vi "Event-Display.vi"(7 "Display":T1(ring), 8 "error in (no error)":errorcluster, 10 "Data ref. in":refnum<data-value>, 11 "UI ref. in":refnum<data-value>) -> (0 "error out":errorcluster, 2 "Data ref.":refnum<data-value>, 3 "UI ref.":refnum<data-value>)   [LabVIEW 2013, in "CameraVision.lvlib" / "CV-UI.lvclass"]
uses:
  CV-UI.lvclass
  Main/CV-Main.lvclass
  CV-UI.lvclass/CV-UI.ctl
  Main/Main-actions.ctl
  Read Display-tab.vi
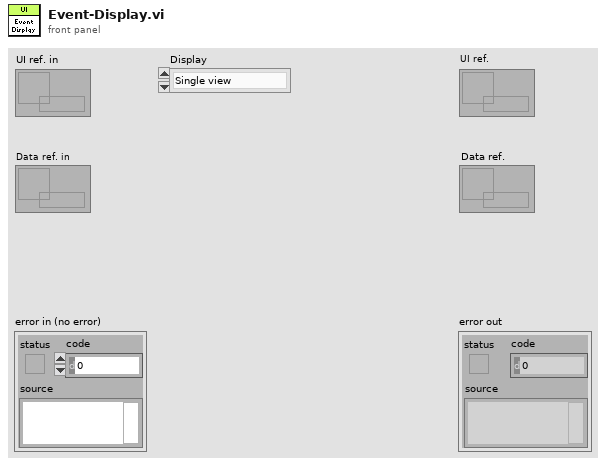
[diagram p1: front panel]
types:
  T1 = enum32{"Single view", "Dual view", "Analysis", "History", "Temperature field", "Mapping", "Debug"}
  T2 = typedef "CameraVision.lvlib/CV-Main.lvclass/Main-actions.ctl" = enum16{"Idle", "Initialize", "Load defaults", "Update settings", "Check settings", "Save settings", "Save settings with dialog", "Load settings", "Load data", "Activate", "Start", "Wait for start signal", "Acquire & process", "Iterate", "Stop", "Refresh display", "Refresh status", "View camera settings", "View grabber settings", "Exit"}
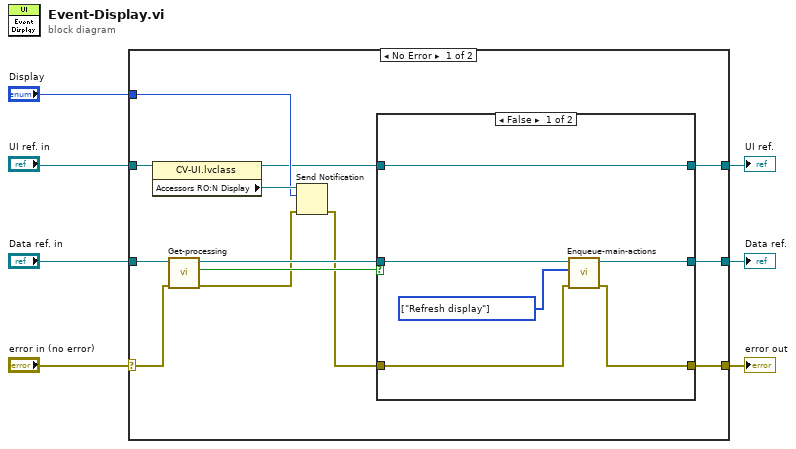
[diagram p0: block diagram]
diagram:
  n1 = case shown="No Error" "error in (no error)" {
    selector: "error in (no error)" -> [w15 w32]
    tunnel: [w14 w32] -> w6
    tunnel: [w17 w31] -> w4
    tunnel: "UI ref. in" -> [w13 w31]
    tunnel: "Data ref. in" -> [w20 w30]
    tunnel: "Display" -> [w9 _]
    tunnel: [w16 w30] -> w2
    frame No Error {
      n2 = property class="CV-UI.lvclass"(reference=w13) -> (reference out=w8:refnum<data-value>, "Accessors RO:N Display"=w12:refnum<notifier>)  [unwired: 1 in, 1 out]
      n3 = call "Get-processing.vi"("error in (no error)"=w15, "Data ref. in"=w20) -> ("error out"=w11:errorcluster, "Processing?"=w18:bool, "Data ref."=w19:refnum<data-value>)  [unwired: 7 in]
      n4 = Send Notification(notification=w9, notifier=w12, error in (no error)=w11) -> (error out=w10:errorcluster)  [unwired: 1 out]
      n5 = case shown="False" w18 {
        tunnel: w8 -> [w23 w28]
        tunnel: w19 -> [w22 w27]
        tunnel: [w23 w28] -> w17
        tunnel: [w21 w27] -> w16
        tunnel: w10 -> [w25 w29]
        tunnel: [w24 w29] -> w14
        frame False {
          w26 = T2[] [enum."Refresh display"] items=["Idle", "Initialize", "Load defaults", "Update settings", "Check settings", "Save settings", "Save settings with dialog", "Load settings", "Load data", "Activate", "Start", "Wait for start signal", "Acquire & process", "Iterate", "Stop", "Refresh display", "Refresh status", "View camera settings", "View grabber settings", "Exit"] ("State array")
          n6 = call "Enqueue-main-actions.vi"("error in (no error)"=w25, "State array"=w26, "Data ref. in"=w22) -> ("error out"=w24:errorcluster, "Data ref."=w21:refnum<data-value>)  [unwired: 6 in, 1 out]
        }
        frame True {
        }
      }
    }
    frame Error {
    }
  }
  "error out" <- w6
  "Data ref." <- w2
  "UI ref." <- w4
